vi "log analysis_gps.vi"() -> ()   [LabVIEW 2018] (continued)
0.0927,0.0768,0.1395,0.1446,5.0385,0f000001,0*5a4f325f\n\tsystem status\tnormal 2 27.900000 0 0\trobot status\t327.041164\t38.648873\t11.416000\t-0.542047\t1.417066\t-27.580040\t0.262000\t0.075000\n\t\n15:26:44.7\tlog_raw\tgps_raw\t#INSPVAXA,USB3,0,52.0,FINESTEERING,2107,282422.700,02000000,471d,15824;INS_ALIGNMENT_COMPLETE,INS_RTKFIXED,37.37047779147,126.72452855561,11.4180,22.3000,-0.1674,0.2510,0.0061,-0.538633427,1.577251598,117.409835923,0.4474,0.2945,0.5457,0.1156,0.0927,0.0768,0.1395,0.1446,5.0385,0f000001,0*702f4b29\n\tsystem status\tnormal 2 28.000000 0 0\trobot status\t327.159797\t38.571286\t11.418000\t-0.538633\t1.577252\t-27.409836\t0.344000\t-0.072000\n\t\n15:26:45.2\tlog_raw\tgps_raw\t#INSPVAXA,USB3,0,53.0,FINESTEERING,2107,282423.200,02000000,471d,15824;INS_ALIGNMENT_COMPLETE,INS_RTKFIXED,37.37047709132,126.72452988330,11.4199,22.3000,-0.1693,0.2361,0.0114,-0.484097590,1.645236384,117.249213535,0.4481,0.2944,0.5459,0.1153,0.0924,0.0769,0.1394,0.1445,5.0397,0f000001,0*1f110da8\n\tsystem status\tnormal 2 28.000000 0 0\trobot status\t327.277401\t38.493575\t11.419900\t-0.484098\t1.645236\t-27.249214\t0.366000\t-0.082000\n\t\n15:26:45.7\tlog_raw\tgps_raw\t#INSPVAXA,USB3,0,53.0,FINESTEERING,2107,282423.700,02000000,471d,15824;INS_ALIGNMENT_COMPLETE,INS_RTKFIXED,37.37047638174,126.72453122858,11.4229,22.3000,-0.1794,0.2589,0.0063,-0.583943678,1.497224393,117.186202901,0.4481,0.2944,0.5459,0.1153,0.0924,0.0769,0.1394,0.1445,5.0397,0f000001,0*d1d8ac53\n\tsystem status\tnormal 2 28.000000 0 0\trobot status\t327.396564\t38.414818\t11.422900\t-0.583944\t1.497224\t-27.186203\t0.298000\t0.020000\n\t\n15:26:46.2\tlog_raw\tgps_raw\t#INSPVAXA,USB3,0,47.5,FINESTEERING,2107,282424.200,02000000,471d,15824;INS_ALIGNMENT_COMPLETE,INS_RTKFIXED,37.37047566683,126.72453256018,11.4256,22.3000,-0.1669,0.2594,-0.0024,-0.470106549,1.538680379,117.122704089,0.4483,0.2943,0.5461,0.1150,0.0923,0.0770,0.1394,0.1445,5.0409,0f000001,0*dc6910b4\n\tsystem status\tnormal 2 28.000000 0 0\trobot status\t327.514515\t38.335469\t11.425600\t-0.470107\t1.538680\t-27.122704\t0.283000\t0.031000\n\t\n15:26:46.7\tlog_raw\tgps_raw\t#INSPVAXA,USB3,0,47.5,FINESTEERING,2107,282424.700,02000000,471d,15824;INS_ALIGNMENT_COMPLETE,INS_RTKFIXED,37.37047494841,126.72453391705,11.4289,22.3000,-0.1673,0.2511,-0.0021,-0.336586213,1.463245271,117.104928251,0.4483,0.2943,0.5461,0.1150,0.0923,0.0770,0.1394,0.1445,5.0409,0f000001,0*1c6dfd0e\n\tsystem status\tnormal 2 28.000000 0 0\trobot status\t327.634704\t38.255731\t11.428900\t-0.336586\t1.463245\t-27.104928\t0.288000\t0.027000\n\t\n15:26:47.2\tlog_raw\tgps_raw\t#INSPVAXA,USB3,0,52.5,FINESTEERING,2107,282425.200,02000000,471d,15824;INS_ALIGNMENT_COMPLETE,INS_RTKFIXED,37.37047424170,126.72453526540,11.4324,22.3000,-0.1767,0.2603,-0.0045,-0.387302146,1.336492111,117.087271319,0.4481,0.2942,0.5464,0.1148,0.0922,0.0770,0.1394,0.1445,5.0421,0f000001,0*5b1ecf9b\n\tsystem status\tnormal 2 28.000000 0 0\trobot status\t327.754139\t38.177293\t11.432400\t-0.387302\t1.336492\t-27.087271\t0.304000\t0.000000\n\t\n15:26:47.7\tlog_raw\tgps_raw\t#INSPVAXA,USB3,0,52.5,FINESTEERING,2107,282425.700,02000000,471d,15824;INS_ALIGNMENT_COMPLETE,INS_RTKFIXED,37.37047353381,126.72453661330,11.4355,22.3000,-0.1756,0.2651,-0.0041,-0.429146495,1.196465105,117.112616572,0.4481,0.2942,0.5464,0.1148,0.0922,0.0770,0.1394,0.1445,5.0421,0f000001,0*c119c68d\n\tsystem status\tnormal 2 28.000000 0 0\trobot status\t327.873534\t38.098723\t11.435500\t-0.429146\t1.196465\t-27.112617\t0.300000\t-0.005000\n\t\n15:26:48.2\tlog_raw\tgps_raw\t#INSPVAXA,USB3,0,49.0,FINESTEERING,2107,282426.200,02000000,471d,15824;INS_ALIGNMENT_COMPLETE,INS_RTKFIXED,37.37047281927,126.72453797131,11.4379,22.3000,-0.1734,0.2394,0.0077,-0.416203988,1.155690665,117.100710288,0.4473,0.2939,0.5465,0.1146,0.0922,0.0771,0.1395,0.1444,5.0432,0f000001,0*775443d5\n\tsystem status\tnormal 2 28.000000 0 0\trobot status\t327.993824\t38.019415\t11.437900\t-0.416204\t1.155691\t-27.100710\t0.298000\t-0.006000\n\t\n15:26:48.7\tlog_raw\tgps_raw\t#INSPVAXA,USB3,0,49.0,FINESTEERING,2107,282426.700,02000000,471d,15824;INS_ALIGNMENT_COMPLETE,INS_RTKFIXED,37.37047210734,126.72453930572,11.4405,22.3000,-0.1867,0.2504,0.0028,-0.209968626,1.098729863,117.099023809,0.4473,0.2939,0.5465,0.1146,0.0922,0.0771,0.1395,0.1444,5.0432,0f000001,0*f26e42b0\n\tsystem status\tnormal 2 28.000000 0 0\trobot status\t328.112024\t37.940397\t11.440500\t-0.209969\t1.098730\t-27.099024\t0.303000\t-0.001000\n\t\n15:26:49.2\tlog_raw\tgps_raw\t#INSPVAXA,USB3,0,49.0,FINESTEERING,2107,282427.200,02000000,471d,15824;INS_ALIGNMENT_COMPLETE,INS_RTKFIXED,37.37047139601,126.72454064039,11.4416,22.3000,-0.1731,0.2492,-0.0012,-0.127511151,0.940148188,117.168833754,0.4465,0.2938,0.5466,0.1144,0.0924,0.0771,0.1395,0.1444,5.0441,0f000001,0*6d877c07\n\tsystem status\tnormal 2 28.000000 0 0\trobot status\t328.230247\t37.861446\t11.441600\t-0.127511\t0.940148\t-27.168834\t0.301000\t-0.007000\n\t\n15:26:49.7\tlog_raw\tgps_raw\t#INSPVAXA,USB3,0,49.0,FINESTEERING,2107,282427.700,02000000,471d,15824;INS_ALIGNMENT_COMPLETE,INS_RTKFIXED,37.37047069525,126.72454194730,11.4442,22.3000,-0.1701,0.2495,0.0012,-0.095196200,0.956873575,117.185221868,0.4465,0.2938,0.5466,0.1144,0.0924,0.0771,0.1395,0.1444,5.0441,0f000001,0*84a20544\n\tsystem status\tnormal 2 28.000000 0 0\trobot status\t328.346010\t37.783668\t11.444200\t-0.095196\t0.956874\t-27.185222\t0.304000\t-0.005000\n\t\n15:26:50.2\tlog_raw\tgps_raw\t#INSPVAXA,USB3,0,48.5,FINESTEERING,2107,282428.200,02000000,471d,15824;INS_ALIGNMENT_COMPLETE,INS_RTKFIXED,37.37046998613,126.72454328070,11.4463,22.3000,-0.1686,0.2345,-0.0007,-0.178803832,1.054572060,117.268598245,0.4452,0.2937,0.5465,0.1143,0.0923,0.0771,0.1395,0.1444,5.0443,0f000001,0*71fff611\n\tsystem status\tnormal 2 28.000000 0 0\trobot status\t328.464121\t37.704962\t11.446300\t-0.178804\t1.054572\t-27.268598\t0.301000\t-0.003000\n\t\n15:26:50.7\tlog_raw\tgps_raw\t#INSPVAXA,USB3,0,48.5,FINESTEERING,2107,282428.700,02000000,471d,15824;INS_ALIGNMENT_COMPLETE,INS_RTKFIXED,37.37046928771,126.72454456958,11.4489,22.3000,-0.1768,0.2502,0.0012,-0.177631825,1.040630154,117.335486579,0.4452,0.2937,0.5465,0.1143,0.0923,0.0771,0.1395,0.1444,5.0443,0f000001,0*5554e59a\n\tsystem status\tnormal 2 28.000000 0 0\trobot status\t328.578288\t37.627444\t11.448900\t-0.177632\t1.040630\t-27.335487\t0.304000\t-0.005000\n\t\n15:26:51.2\tlog_raw\tgps_raw\t#INSPVAXA,USB3,0,50.5,FINESTEERING,2107,282429.200,02000000,471d,15824;INS_ALIGNMENT_COMPLETE,INS_RTKFIXED,37.37046858218,126.72454587294,11.4510,22.3000,-0.1735,0.2382,-0.0057,-0.224101923,1.178682503,117.429703451,0.4445,0.2937,0.5467,0.1141,0.0923,0.0771,0.1395,0.1444,5.0440,0f000001,0*7240883e\n\tsystem status\tnormal 2 28.000000 0 0\trobot status\t328.693737\t37.549136\t11.451000\t-0.224102\t1.178683\t-27.429703\t0.303000\t-0.014000\n\t\n15:26:51.7\tlog_raw\tgps_raw\t#INSPVAXA,USB3,0,50.5,FINESTEERING,2107,282429.700,02000000,471d,15824;INS_ALIGNMENT_COMPLETE,INS_RTKFIXED,37.37046786468,126.72454718856,11.4534,22.3000,-0.1761,0.2406,-0.0007,-0.208083401,1.502280948,117.509973758,0.4445,0.2937,0.5467,0.1141,0.0923,0.0771,0.1395,0.1444,5.0440,0f000001,0*e6f82928\n\tsystem status\tnormal 2 28.000000 0 0\trobot status\t328.810273\t37.469500\t11.453400\t-0.208083\t1.502281\t-27.509974\t0.294000\t-0.015000\n\t\n15:26:52.2\tlog_raw\tgps_raw\t#INSPVAXA,USB3,0,50.5,FINESTEERING,2107,282430.200,02000000,471d,15824;INS_ALIGNMENT_COMPLETE,INS_RTKFIXED,37.37046713454,126.72454853223,11.4571,22.3000,-0.1871,0.2437,0.0106,-0.235134263,1.524805783,117.657150999,0.4436,0.2937,0.5464,0.1140,0.0923,0.0770,0.1395,0.1444,5.0440,0f000001,0*40fb5b15\n\tsystem status\tnormal 2 28.000000 0 0\trobot status\t328.929293\t37.388461\t11.457100\t-0.235134\t1.524806\t-27.657151\t0.302000\t-0.003000\n\t\n15:26:52.7\tlog_raw\tgps_raw\t#INSPVAXA,USB3,0,50.5,FINESTEERING,2107,282430.700,02000000,471d,15824;INS_ALIGNMENT_COMPLETE,INS_RTKFIXED,37.37046640925,126.72454987215,11.4613,22.3000,-0.1820,0.2459,0.0096,-0.221423575,1.571464765,117.878951435,0.4436,0.2937,0.5464,0.1140,0.0923,0.0770,0.1395,0.1444,5.0440,0f000001,0*a08ac800\n\tsystem status\tnormal 2 28.000000 0 0\trobot status\t329.047981\t37.307960\t11.461300\t-0.221424\t1.571465\t-27.878951\t0.302000\t-0.009000\n\t\n15:26:53.2\tlog_raw\tgps_raw\t#INSPVAXA,USB3,0,50.5,FINESTEERING,2107,282431.200,02000000,471d,15824;INS_ALIGNMENT_COMPLETE,INS_RTKFIXED,37.37046567554,126.72455119637,11.4651,22.3000,-0.1719,0.2427,0.0197,-0.166037834,1.730159075,118.106300451,0.4429,0.2934,0.5460,0.1140,0.0922,0.0770,0.1395,0.1444,5.0446,0f000001,0*c5fa0f53\n\tsystem status\tnormal 2 28.000000 0 0\trobot status\t329.165278\t37.226525\t11.465100\t-0.166038\t1.730159\t-28.106300\t0.300000\t-0.008000\n\t\n15:26:53.7\tlog_raw\tgps_raw\t#INSPVAXA,USB3,0,50.5,FINESTEERING,2107,282431.700,02000000,471d,15824;INS_ALIGNMENT_COMPLETE,INS_RTKFIXED,37.37046493957,126.72455254233,11.4688,22.3000,-0.1743,0.2458,0.0116,-0.329831590,1.590746400,118.317737739,0.4429,0.2934,0.5460,0.1140,0.0922,0.0770,0.1395,0.1444,5.0446,0f000001,0*f79436a0\n\tsystem status\tnormal 2 28.000000 0 0\trobot status\t329.284501\t37.144839\t11.468800\t-0.329832\t1.590746\t-28.317738\t0.295000\t-0.010000\n\t\n15:26:54.2\tlog_raw\tgps_raw\t#INSPVAXA,USB3,0,51.5,FINESTEERING,2107,282432.200,02000000,471d,15824;INS_ALIGNMENT_COMPLETE,INS_RTKFIXED,37.37046419639,126.72455389364,11.4732,22.3000,-0.1776,0.2446,0.0108,-0.495947229,1.503105474,118.571137499,0.4424,0.2936,0.5455,0.1139,0.0922,0.0769,0.1394,0.1444,5.0458,0f000001,0*be714efa\n\tsystem status\tnormal 2 28.000000 0 0\trobot status\t329.404198\t37.062353\t11.473200\t-0.495947\t1.503105\t-28.571137\t0.296000\t-0.015000\n\t\n15:26:54.7\tlog_raw\tgps_raw\t#INSPVAXA,USB3,0,51.5,FINESTEERING,2107,282432.700,02000000,471d,15824;INS_ALIGNMENT_COMPLETE,INS_RTKFIXED,37.37046345455,126.72455522466,11.4784,22.3000,-0.1781,0.2428,0.0084,-0.542024872,1.613123448,118.821399108,0.4424,0.2936,0.5455,0.1139,0.0922,0.0769,0.1394,0.1444,5.0458,0f000001,0*f6f3aed6\n\tsystem status\tnormal 2 28.000000 0 0\trobot status\t329.522097\t36.980016\t11.478400\t-0.542025\t1.613123\t-28.821399\t0.295000\t-0.017000\n\t\n15:26:55.2\tlog_raw\tgps_raw\t#INSPVAXA,USB3,0,50.0,FINESTEERING,2107,282433.200,02000000,471d,15824;INS_ALIGNMENT_COMPLETE,INS_RTKFIXED,37.37046270348,126.72455655878,11.4838,22.3000,-0.1795,0.2457,0.0085,-0.467602875,1.636327980,119.061626525,0.4415,0.2938,0.5451,0.1139,0.0923,0.0769,0.1394,0.1444,5.0472,0f000001,0*8d27345e\n\tsystem status\tnormal 2 28.000000 0 0\trobot status\t329.640271\t36.896654\t11.483800\t-0.467603\t1.636328\t-29.061627\t0.302000\t-0.014000\n\t\n15:26:55.7\tlog_raw\tgps_raw\t#DUALANTENNAHEADINGA,USB3,0,50.0,FINESTEERING,2107,282433.700,02000000,d426,15824;SOL_COMPUTED,NARROW_FLOAT,-1.000000000,131.824783325,-60.644287109,0.0,360.000000000,180.000000000,\"631T\",16,7,7,6,04,00,20,03*5e82c6fa\n\tsystem status\tnormal 2 28.000000 0 0\trobot status\t329.757799\t36.814629\t11.489300\t-0.433063\t1.678880\t-29.334865\t0.303000\t-0.012000\n\t\n15:26:56.2\tlog_raw\tgps_raw\t#INSPVAXA,USB3,0,51.0,FINESTEERING,2107,282434.200,02000000,471d,15824;INS_ALIGNMENT_COMPLETE,INS_RTKFIXED,37.37046121342,126.72455921489,11.4947,22.3000,-0.1798,0.2490,0.0001,-0.438174613,1.842528382,119.643730072,0.4410,0.2940,0.5447,0.1139,0.0923,0.0769,0.1394,0.1443,5.0488,0f000001,0*2736b416\n\tsystem status\tnormal 2 28.000000 0 0\trobot status\t329.875545\t36.731271\t11.494700\t-0.438175\t1.842528\t-29.643730\t0.309000\t-0.015000\n\t\n15:26:56.7\tlog_raw\tgps_raw\t#DUALANTENNAHEADINGA,USB3,0,51.0,FINESTEERING,2107,282434.700,02000000,d426,15824;SOL_COMPUTED,NARROW_FLOAT,-1.000000000,123.396003723,-59.946563721,0.0,360.000000000,180.000000000,\"631T\",18,7,7,6,04,00,20,03*e2309186\n\tsystem status\tnormal 2 28.000000 0 0\trobot status\t329.993174\t36.646447\t11.500400\t-0.411549\t1.662187\t-29.943410\t0.300000\t-0.011000\n\t\n15:26:57.2\tlog_raw\tgps_raw\t#INSPVAXA,USB3,0,52.0,FINESTEERING,2107,282435.200,02000000,471d,15824;INS_ALIGNMENT_COMPLETE,INS_RTKFIXED,37.37045967232,126.72456187341,11.5062,22.3000,-0.1775,0.2335,0.0126,-0.320080910,1.572819973,120.246717938,0.4403,0.2940,0.5441,0.1137,0.0923,0.0768,0.1394,0.1443,5.0504,0f000001,0*2715df5d\n\tsystem status\tnormal 2 28.000000 0 0\trobot status\t330.111033\t36.560223\t11.506200\t-0.320081\t1.572820\t-30.246718\t0.290000\t-0.019000\n\t\n15:26:57.7\tlog_raw\tgps_raw\t#INSPVAXA,USB3,0,52.0,FINESTEERING,2107,282435.700,02000000,471d,15824;INS_ALIGNMENT_COMPLETE,INS_RTKFIXED,37.37045891592,126.72456315232,11.5133,22.3000,-0.1801,0.2388,0.0143,-0.294831475,1.595184630,120.686846518,0.4403,0.2940,0.5441,0.1137,0.0923,0.0768,0.1394,0.1443,5.0504,0f000001,0*d40acedf\n\tsystem status\tnormal 2 28.000000 0 0\trobot status\t330.224316\t36.476270\t11.513300\t-0.294831\t1.595185\t-30.686847\t0.300000\t-0.018000\n\t\n15:26:58.2\tlog_raw\tgps_raw\t#DUALANTENNAHEADINGA,USB3,0,49.0,FINESTEERING,2107,282436.200,02000000,d426,15824;SOL_COMPUTED,L1_FLOAT,-1.000000000,106.640296936,-71.318817139,0.0,360.000000000,180.000000000,\"631T\",16,6,6,6,04,00,20,02*b4f0dd4d\n\tsystem status\tnormal 2 28.000000 0 0\trobot status\t330.338646\t36.390312\t11.520900\t-0.272505\t1.410764\t-31.156863\t0.335000\t0.034000\n\t\n15:26:58.7\tlog_raw\tgps_raw\t#INSPVAXA,USB3,0,49.0,FINESTEERING,2107,282436.700,02000000,471d,15824;INS_ALIGNMENT_COMPLETE,INS_RTKFIXED,37.37045734595,126.72456573410,11.5280,22.3000,-0.1935,0.2298,0.0134,-0.155063449,1.404576364,121.642005651,0.4395,0.2941,0.5437,0.1137,0.0923,0.0768,0.1394,0.1443,5.0520,0f000001,0*bb2e31e4\n\tsystem status\tnormal 2 28.000000 0 0\trobot status\t330.453006\t36.302018\t11.528000\t-0.155063\t1.404576\t-31.642006\t0.365000\t0.096000\n\t\n15:26:59.2\tlog_raw\tgps_raw\t#DUALANTENNAHEADINGA,USB3,0,50.0,FINESTEERING,2107,282437.200,02000000,d426,15824;SOL_COMPUTED,L1_FLOAT,-1.000000000,96.910743713,-72.679077148,0.0,360.000000000,180.000000000,\"631T\",19,6,6,6,04,00,20,02*8360ff91\n\tsystem status\tnormal 2 28.000000 0 0\trobot status\t330.566267\t36.213333\t11.534500\t-0.164952\t1.430283\t-32.232703\t0.293000\t-0.018000\n\t\n15:26:59.7\tlog_raw\tgps_raw\t#INSPVAXA,USB3,0,50.0,FINESTEERING,2107,282437.700,02000000,471d,15824;INS_ALIGNMENT_COMPLETE,INS_RTKFIXED,37.37045573344,126.72456827532,11.5401,22.3000,-0.1925,0.2230,0.0039,-0.101664053,1.395103847,122.819960781,0.4390,0.2940,0.5434,0.1136,0.0923,0.0768,0.1393,0.1443,5.0536,0f000001,0*7037bf1b\n\tsystem status\tnormal 2 28.000000 0 0\trobot status\t330.678103\t36.123046\t11.540100\t-0.101664\t1.395104\t-32.819961\t0.253000\t-0.080000\n\t\n15:27:00.2\tlog_raw\tgps_raw\t#INSPVAXA,USB3,0,50.0,FINESTEERING,2107,282438.200,02000000,471d,15824;INS_ALIGNMENT_COMPLETE,INS_RTKFIXED,37.37045491060,126.72456953243,11.5455,22.3000,-0.2008,0.2357,0.0053,0.014344275,1.355437453,123.346628191,0.4390,0.2941,0.5434,0.1137,0.0924,0.0768,0.1393,0.1442,5.0551,0f000001,0*dff132ba\n\tsystem status\tnormal 2 28.000000 0 0\trobot status\t330.789456\t36.031719\t11.545500\t0.014344\t1.355437\t-33.346628\t0.238000\t-0.107000\n\t\n15:27:00.7\tlog_raw\tgps_raw\t#DUALANTENNAHEADINGA,USB3,0,50.0,FINESTEERING,2107,282438.700,02000000,d426,15824;SOL_COMPUTED,L1_FLOAT,-1.000000000,88.413047791,-71.788269043,0.0,360.000000000,180.000000000,\"631T\",18,6,6,6,04,00,20,02*2c629dff\n\tsystem status\tnormal 2 28.000000 0 0\trobot status\t330.900070\t35.941719\t11.550100\t-0.061999\t1.261204\t-33.976038\t0.479000\t0.250000\n\t\n15:27:01.2\tlog_raw\tgps_raw\t#INSPVAXA,USB3,0,50.0,FINESTEERING,2107,282439.200,02000000,471d,15824;INS_ALIGNMENT_COMPLETE,INS_RTKFIXED,37.37045327515,126.72457200687,11.5547,22.3000,-0.1947,0.2312,0.0176,0.007839665,1.196473150,124.504878880,0.4394,0.2943,0.5435,0.1138,0.0925,0.0768,0.1393,0.1442,5.0565,0f000001,0*62131131\n\tsystem status\tnormal 2 28.000000 0 0\trobot status\t331.008638\t35.850200\t11.554700\t0.007840\t1.196473\t-34.504879\t0.366000\t0.072000\n\t\n15:27:01.7\tlog_raw\tgps_raw\t#INSPVAXA,USB3,0,50.0,FINESTEERING,2107,282439.700,02000000,471d,15824;INS_ALIGNMENT_COMPLETE,INS_RTKFIXED,37.37045245095,126.72457319458,11.5591,22.3000,-0.1909,0.2308,0.0250,0.014196005,1.345300679,124.975912941,0.4394,0.2943,0.5435,0.1138,0.0925,0.0768,0.1393,0.1442,5.0565,0f000001,0*c01a2c95\n\tsystem status\tnormal 2 28.000000 0 0\trobot status\t331.113843\t35.758723\t11.559100\t0.014196\t1.345301\t-34.975913\t0.284000\t-0.034000\n\t\n15:27:02.2\tlog_raw\tgps_raw\t#DUALANTENNAHEADINGA,USB3,0,50.5,FINESTEERING,2107,282440.200,02000000,d426,15824;SOL_COMPUTED,L1_FLOAT,-1.000000000,104.733528137,-71.981353760,0.0,360.000000000,180.000000000,\"631T\",16,6,6,6,04,00,20,02*496cf2b0\n\tsystem status\tnormal 2 28.000000 0 0\trobot status\t331.219713\t35.666735\t11.563700\t0.016944\t1.696880\t-35.321999\t0.302000\t-0.004000\n\t\n15:27:02.7\tlog_raw\tgps_raw\t#INSPVAXA,USB3,0,50.5,FINESTEERING,2107,282440.700,02000000,471d,15824;INS_ALIGNMENT_COMPLETE,INS_RTKFIXED,37.37045078135,126.72457562131,11.5665,22.3000,-0.1912,0.2138,0.0152,-0.119688285,1.522549253,125.693506579,0.4396,0.2937,0.5434,0.1139,0.0925,0.0768,0.1392,0.1442,5.0578,0f000001,0*ce1f2ed1\n\tsystem status\tnormal 2 28.000000 0 0\trobot status\t331.328799\t35.573414\t11.566500\t-0.119688\t1.522549\t-35.693507\t0.344000\t0.082000\n\t\n15:27:03.2\tlog_raw\tgps_raw\t#DUALANTENNAHEADINGA,USB3,0,53.0,FINESTEERING,2107,282441.200,02000000,d426,15824;SOL_COMPUTED,L1_FLOAT,-1.000000000,98.119506836,-70.068420410,0.0,360.000000000,180.000000000,\"631T\",15,6,6,6,04,00,20,02*34737370\n\tsystem status\tnormal 2 28.000000 0 0\trobot status\t331.432619\t35.480504\t11.569000\t-0.082738\t1.498113\t-36.012425\t0.247000\t-0.082000\n\t\n15:27:03.7\tlog_raw\tgps_raw\t#INSPVAXA,USB3,0,53.0,FINESTEERING,2107,282441.700,02000000,471d,15824;INS_ALIGNMENT_COMPLETE,INS_RTKFIXED,37.37044907161,126.72457798223,11.5726,22.3000,-0.1948,0.2179,0.0112,0.019648441,1.409240811,126.353403085,0.4397,0.2935,0.5431,0.1139,0.0925,0.0768,0.1391,0.1441,5.0591,0f000001,0*4c7348f3\n\tsystem status\tnormal 2 28.000000 0 0\trobot status\t331.537926\t35.383651\t11.572600\t0.019648\t1.409241\t-36.353403\t0.229000\t-0.093000\n\t\n15:27:04.2\tlog_raw\tgps_raw\t#DUALANTENNAHEADINGA,USB3,0,53.0,FINESTEERING,2107,282442.200,02000000,d426,15824;SOL_COMPUTED,L1_FLOAT,-1.000000000,135.735549927,-62.905853271,0.0,360.000000000,180.000000000,\"631T\",15,6,6,6,04,00,20,02*7d1a323e\n\tsystem status\tnormal 2 28.000000 0 0\trobot status\t331.643745\t35.286306\t11.577800\t0.040624\t1.148557\t-36.777461\t0.347000\t0.059000\n\t\n15:27:04.7\tlog_raw\tgps_raw\t#DUALANTENNAHEADINGA,USB3,0,53.0,FINESTEERING,2107,282442.700,02000000,d426,15824;SOL_COMPUTED,L1_FLOAT,-1.000000000,139.850036621,-63.364013672,0.0,360.000000000,180.000000000,\"631T\",16,6,6,6,04,00,20,02*201824d6\n\tsystem status\tnormal 2 28.000000 0 0\trobot status\t331.748506\t35.190562\t11.582000\t-0.114390\t1.160307\t-37.256257\t0.280000\t-0.049000\n\t\n15:27:05.2\tlog_raw\tgps_raw\t#INSPVAXA,USB3,0,51.0,FINESTEERING,2107,282443.200,02000000,471d,15824;INS_ALIGNMENT_COMPLETE,INS_RTKFIXED,37.37044646413,126.72458151712,11.5864,22.3000,-0.1973,0.2015,0.0164,-0.221608077,1.394071169,127.627895652,0.4382,0.2942,0.5425,0.1139,0.0929,0.0768,0.1390,0.1440,5.0619,0f000001,0*d0821dfc\n\tsystem status\tnormal 2 28.000000 0 0\trobot status\t331.851040\t35.094249\t11.586400\t-0.221608\t1.394071\t-37.627896\t0.338000\t0.046000\n\t\n15:27:05.7\tlog_raw\tgps_raw\t#DUALANTENNAHEADINGA,USB3,0,51.0,FINESTEERING,2107,282443.700,02000000,d426,15824;SOL_COMPUTED,NARROW_FLOAT,-1.000000000,112.599952698,-57.933044434,0.0,360.000000000,180.000000000,\"631T\",15,6,6,6,04,00,20,03*0a41350b\n\tsystem status\tnormal 2 28.000000 0 0\trobot status\t331.952897\t34.994891\t11.593000\t-0.249153\t1.572965\t-38.005093\t0.379000\t0.102000\n\t\n15:27:06.2\tlog_raw\tgps_raw\t#DUALANTENNAHEADINGA,USB3,0,52.5,FINESTEERING,2107,282444.200,02000000,d426,15824;SOL_COMPUTED,L1_FLOAT,-1.000000000,94.401931763,-65.202850342,0.0,360.000000000,180.000000000,\"631T\",17,6,6,6,04,00,20,03*e210f1e8\n\tsystem status\tnormal 2 28.000000 0 0\trobot status\t332.052872\t34.895652\t11.599300\t-0.212433\t1.862768\t-38.371437\t0.256000\t-0.080000\n\t\n15:27:06.7\tlog_raw\tgps_raw\t#INSPVAXA,USB3,0,52.5,FINESTEERING,2107,282444.700,02000000,471d,15824;INS_ALIGNMENT_COMPLETE,INS_RTKFIXED,37.37044378367,126.72458489519,11.6040,22.3000,-0.1971,0.2104,0.0118,-0.197880099,2.000562987,128.752453378,0.4375,0.2942,0.5421,0.1140,0.0930,0.0767,0.1389,0.1439,5.0634,0f000001,0*c33b9934\n\tsystem status\tnormal 2 28.000000 0 0\trobot status\t332.150264\t34.796747\t11.604000\t-0.197880\t2.000563\t-38.752453\t0.332000\t0.027000\n\t\n15:27:07.2\tlog_raw\tgps_raw\t#INSPVAXA,USB3,0,52.0,FINESTEERING,2107,282445.200,02000000,471d,15824;INS_ALIGNMENT_COMPLETE,INS_RTKFIXED,37.37044286692,126.72458603367,11.6088,22.3000,-0.1958,0.2105,0.0125,-0.182257004,1.882197193,129.119511082,0.4372,0.2942,0.5419,0.1140,0.0930,0.0767,0.1387,0.1438,5.0651,0f000001,0*e6286548\n\tsystem status\tnormal 2 28.000000 0 0\trobot status\t332.251109\t34.694998\t11.608800\t-0.182257\t1.882197\t-39.119511\t0.284000\t-0.033000\n\t\n15:27:07.7\tlog_raw\tgps_raw\t#INSPVAXA,USB3,0,52.0,FINESTEERING,2107,282445.700,02000000,471d,15824;INS_ALIGNMENT_COMPLETE,INS_RTKFIXED,37.37044196596,126.72458716165,11.6139,22.3000,-0.1860,0.1986,0.0135,-0.288793449,1.691261499,129.571848658,0.4372,0.2942,0.5419,0.1140,0.0930,0.0767,0.1387,0.1438,5.0651,0f000001,0*93ea3f3c\n\tsystem status\tnormal 2 28.000000 0 0\trobot status\t332.351024\t34.595001\t11.613900\t-0.288793\t1.691261\t-39.571849\t0.238000\t-0.092000\n\t\n15:27:08.2\tlog_raw\tgps_raw\t#INSPVAXA,USB3,0,49.5,FINESTEERING,2107,282446.200,02000000,471d,15824;INS_ALIGNMENT_COMPLETE,INS_RTKFIXED,37.37044104802,126.72458827290,11.6191,22.3000,-0.2036,0.2086,0.0326,-0.314944845,1.597002545,130.029060418,0.4370,0.2950,0.5417,0.1141,0.0931,0.0767,0.1386,0.1437,5.0666,0f000001,0*166a3618\n\tsystem status\tnormal 2 28.000000 0 0\trobot status\t332.449456\t34.493120\t11.619100\t-0.314945\t1.597003\t-40.029060\t0.265000\t-0.068000\n\t\n15:27:08.7\tlog_raw\tgps_raw\t#DUALANTENNAHEADINGA,USB3,0,49.5,FINESTEERING,2107,282446.700,02000000,d426,15824;SOL_COMPUTED,L1_FLOAT,-1.000000000,72.571334839,-68.740661621,0.0,360.000000000,180.000000000,\"631T\",16,6,6,6,04,00,20,02*f8abca53\n\tsystem status\tnormal 2 28.000000 0 0\trobot status\t332.546590\t34.388271\t11.623500\t-0.257290\t1.459465\t-40.450598\t0.287000\t-0.037000\n\t\n15:27:09.2\tlog_raw\tgps_raw\t#DUALANTENNAHEADINGA,USB3,0,51.0,FINESTEERING,2107,282447.200,02000000,d426,15824;SOL_COMPUTED,L1_FLOAT,-1.000000000,47.042289734,-21.824493408,0.0,80.520454407,171.226654053,\"631T\",17,6,6,6,04,00,20,02*c2df237f\n\tsystem status\tnormal 2 28.000000 0 0\trobot status\t332.644198\t34.281714\t11.627900\t-0.223387\t1.426203\t-40.898796\t0.297000\t-0.021000\n\t\n15:27:09.7\tlog_raw\tgps_raw\t#DUALANTENNAHEADINGA,USB3,0,51.0,FINESTEERING,2107,282447.700,02000000,d426,15824;SOL_COMPUTED,L1_FLOAT,-1.000000000,47.179916382,-22.115081787,0.0,81.568397522,172.185485840,\"631T\",16,6,6,6,04,00,20,02*ed165946\n\tsystem status\tnormal 2 28.000000 0 0\trobot status\t332.740064\t34.175121\t11.632300\t-0.181305\t1.536050\t-41.293429\t0.230000\t-0.140000\n\t\n15:27:10.2\tlog_raw\tgps_raw\t#DUALANTENNAHEADINGA,USB3,0,50.0,FINESTEERING,2107,282448.200,02000000,d426,15824;SOL_COMPUTED,L1_FLOAT,-1.000000000,62.731056213,-70.065948486,0.0,206.330291748,71.296012878,\"631T\",14,6,6,6,04,00,20,02*363416aa\n\tsystem status\tnormal 2 28.000000 0 0\trobot status\t332.834657\t34.068208\t11.636100\t-0.115686\t1.476151\t-41.714557\t0.390000\t0.115000\n\t\n15:27:10.7\tlog_raw\tgps_raw\t#DUALANTENNAHEADINGA,USB3,0,50.0,FINESTEERING,2107,282448.700,02000000,d426,15824;SOL_COMPUTED,L1_FLOAT,-1.000000000,63.022411346,-70.363861084,0.0,209.852844238,71.028411865,\"631T\",14,6,6,6,04,00,20,02*916b79b1\n\tsystem status\tnormal 2 28.000000 0 0\trobot status\t332.929227\t33.960423\t11.639600\t-0.032914\t1.412595\t-42.067296\t0.272000\t-0.049000\n\t\n15:27:11.2\tlog_raw\tgps_raw\t#INSPVAXA,USB3,0,52.0,FINESTEERING,2107,282449.200,02000000,471d,15824;INS_ALIGNMENT_COMPLETE,INS_RTKFIXED,37.37043526808,126.72459474033,11.6436,22.3000,-0.2045,0.1792,0.0240,0.090566175,1.487884690,132.369305266,0.4363,0.2959,0.5410,0.1143,0.0932,0.0767,0.1382,0.1433,5.0710,0f000001,0*e0923cb2\n\tsystem status\tnormal 2 28.000000 0 0\trobot status\t333.022331\t33.851613\t11.643600\t0.090566\t1.487885\t-42.369305\t0.345000\t0.066000\n\t\n15:27:11.7\tlog_raw\tgps_raw\t#DUALANTENNAHEADINGA,USB3,0,52.0,FINESTEERING,2107,282449.700,02000000,d426,15824;SOL_COMPUTED,L1_FLOAT,-1.000000000,47.736373901,-41.870452881,0.0,87.065238953,101.863716125,\"631T\",13,6,6,6,04,00,20,02*14df9d16\n\tsystem status\tnormal 2 28.000000 0 0\trobot status\t333.114293\t33.743890\t11.647700\t0.044999\t1.426997\t-42.670199\t0.294000\t-0.011000\n\t\n15:27:12.2\tlog_raw\tgps_raw\t#DUALANTENNAHEADINGA,USB3,0,53.5,FINESTEERING,2107,282450.200,02000000,d426,15824;SOL_COMPUTED,L1_FLOAT,-1.000000000,51.328735352,-27.176086426,0.0,71.032249451,148.623870850,\"631T\",13,6,6,6,04,00,20,02*70d3e876\n\tsystem status\tnormal 2 28.000000 0 0\trobot status\t333.205049\t33.634125\t11.650600\t0.240136\t1.430661\t-42.939350\t0.307000\t-0.007000\n\t\n15:27:12.7\tlog_raw\tgps_raw\t#DUALANTENNAHEADINGA,USB3,0,53.5,FINESTEERING,2107,282450.700,02000000,d426,15824;SOL_COMPUTED,L1_FLOAT,-1.000000000,51.277191162,-27.081176758,0.0,70.920402527,148.848937988,\"631T\",13,6,6,6,04,00,20,02*7b58cb2d\n\tsystem status\tnormal 2 28.000000 0 0\trobot status\t333.298460\t33.521084\t11.652900\t0.368602\t1.372850\t-43.254713\t0.294000\t-0.011000\n\t\n15:27:13.2\tlog_raw\tgps_raw\t#DUALANTENNAHEADINGA,USB3,0,52.5,FINESTEERING,2107,282451.200,02000000,d426,15824;SOL_COMPUTED,L1_FLOAT,-1.000000000,57.890838623,-57.911682129,0.0,124.624069214,87.193580627,\"631T\",15,6,6,6,04,00,20,02*079d44e7\n\tsystem status\tnormal 2 28.000000 0 0\trobot status\t333.389705\t33.410958\t11.655500\t0.274163\t1.507707\t-43.538741\t0.296000\t-0.007000\n\t\n15:27:13.7\tlog_raw\tgps_raw\t#DUALANTENNAHEADINGA,USB3,0,52.5,FINESTEERING,2107,282451.700,02000000,d426,15824;SOL_COMPUTED,L1_FLOAT,-1.000000000,57.663475037,-57.904479980,0.0,124.210479736,87.412086487,\"631T\",14,6,6,6,04,00,20,03*cca5b843\n\tsystem status\tnormal 2 28.000000 0 0\trobot status\t333.482165\t33.298901\t11.658400\t0.177384\t1.428253\t-43.810446\t0.296000\t-0.012000\n\t\n15:27:14.2\tlog_raw\tgps_raw\t#DUALANTENNAHEADINGA,USB3,0,52.0,FINESTEERING,2107,282452.200,02000000,d426,15824;SOL_COMPUTED,L1_FLOAT,-1.000000000,54.869430542,-44.105773926,0.0,97.000511169,118.565223694,\"631T\",14,6,6,6,04,00,20,02*875da1f2\n\tsystem status\tnormal 2 28.000000 0 0\trobot status\t333.573111\t33.186729\t11.660700\t0.187302\t1.410985\t-44.065241\t0.300000\t-0.010000\n\t\n15:27:14.7\tlog_raw\tgps_raw\t#DUALANTENNAHEADINGA,USB3,0,52.0,FINESTEERING,2107,282452.700,02000000,d426,15824;SOL_COMPUTED,L1_FLOAT,-1.000000000,55.240604401,-44.770904541,0.0,98.983810425,117.544937134,\"631T\",14,6,6,6,04,00,20,02*e9f54d5e\n\tsystem status\tnormal 2 28.000000 0 0\trobot status\t333.662065\t33.075313\t11.662300\t0.284712\t1.506154\t-44.271764\t0.300000\t0.003000\n\t\n15:27:15.2\tlog_raw\tgps_raw\t#DUALANTENNAHEADINGA,USB3,0,50.5,FINESTEERING,2107,282453.200,02000000,d426,15824;SOL_COMPUTED,L1_FLOAT,-1.000000000,53.051345825,-30.869628906,0.0,85.964683533,159.088867188,\"631T\",12,6,6,6,04,00,20,02*9757b4ba\n\tsystem status\tnormal 2 28.000000 0 0\trobot status\t333.749907\t32.964151\t11.664300\t0.398079\t1.550212\t-44.520288\t0.304000\t-0.002000\n\t\n15:27:15.7\tlog_raw\tgps_raw\t#DUALANTENNAHEADINGA,USB3,0,50.5,FINESTEERING,2107,282453.700,02000000,d426,15824;SOL_COMPUTED,L1_FLOAT,-1.000000000,53.156692505,-31.481872559,0.0,86.806381226,157.845855713,\"631T\",12,6,6,6,04,00,20,02*cbe10416\n\tsystem status\tnormal 2 28.000000 0 0\trobot status\t333.838695\t32.853047\t11.667600\t0.324248\t1.452403\t-44.787555\t0.299000\t-0.003000\n\t\n15:27:16.2\tlog_raw\tgps_raw\t#DUALANTENNAHEADINGA,USB3,0,52.0,FINESTEERING,2107,282454.200,02000000,d426,15824;SOL_COMPUTED,L1_FLOAT,-1.000000000,52.780334473,-53.877258301,0.0,130.208221436,141.251815796,\"631T\",14,6,6,6,04,00,20,02*fcced73a\n\tsystem status\tnormal 2 28.000000 0 0\trobot status\t333.930474\t32.739277\t11.670000\t0.290150\t1.254826\t-44.992673\t0.300000\t0.000000\n\t\n15:27:16.7\tlog_raw\tgps_raw\t#DUALANTENNAHEADINGA,USB3,0,52.0,FINESTEERING,2107,282454.700,02000000,d426,15824;SOL_COMPUTED,L1_FLOAT,-1.000000000,52.636894226,-53.647705078,0.0,129.656005859,142.158767700,\"631T\",13,6,6,6,04,00,20,02*0d3c93fe\n\tsystem status\tnormal 2 28.000000 0 0\trobot status\t334.021378\t32.628145\t11.671800\t0.255531\t1.219635\t-45.071871\t0.297000\t0.001000\n\t\n15:27:17.2\tlog_raw\tgps_raw\t\tsystem status\tnormal 2 28.000000 0 0\trobot status\t334.114386\t32.514788\t11.673700\t0.196509\t1.072827\t-45.139294\t0.294000\t0.012000\n\t\n15:27:17.7\tlog_raw\tgps_raw\t#DUALANTENNAHEADINGA,USB3,0,51.5,FINESTEERING,2107,282455.700,02000000,d426,15824;SOL_COMPUTED,L1_FLOAT,-1.000000000,51.760696411,-51.082702637,0.0,133.844039917,173.444122314,\"631T\",14,6,6,6,04,00,20,02*f8aac9e6\n\tsystem status\tnormal 2 28.000000 0 0\trobot status\t334.206369\t32.399036\t11.675200\t0.326858\t0.794167\t-45.162591\t0.295000\t0.004000\n\t\n15:27:18.2\tlog_raw\tgps_raw\t#DUALANTENNAHEADINGA,USB3,0,53.5,FINESTEERING,2107,282456.200,02000000,d426,15824;SOL_COMPUTED,L1_FLOAT,-1.000000000,51.028530121,-49.821136475,0.0,115.512840271,104.671615601,\"631T\",14,6,6,6,04,00,20,02*e59d7854\n\tsystem status\tnormal 2 28.000000 0 0\trobot status\t334.298520\t32.282316\t11.675800\t0.467199\t0.679863\t-45.205921\t0.299000\t0.005000\n\t\n15:27:18.7\tlog_raw\tgps_raw\t#DUALANTENNAHEADINGA,USB3,0,53.5,FINESTEERING,2107,282456.700,02000000,d426,15824;SOL_COMPUTED,L1_FLOAT,-1.000000000,51.237274170,-50.023620605,0.0,116.616584778,104.545890808,\"631T\",13,6,6,6,04,00,20,02*1b2f8a7d\n\tsystem status\tnormal 2 28.000000 0 0\trobot status\t334.388515\t32.167668\t11.676700\t0.570279\t0.764132\t-45.179052\t0.300000\t0.008000\n\t\n15:27:19.2\tlog_raw\tgps_raw\t#DUALANTENNAHEADINGA,USB3,0,53.0,FINESTEERING,2107,282457.200,02000000,d426,15824;SOL_COMPUTED,L1_FLOAT,-1.000000000,50.694931030,-44.774475098,0.0,121.998092651,121.907302856,\"631T\",13,6,6,6,04,00,20,02*d464c5aa\n\tsystem status\tnormal 2 28.000000 0 0\trobot status\t334.479714\t32.052386\t11.679100\t0.588296\t0.790634\t-45.211656\t0.303000\t0.014000\n\t\n15:27:19.7\tlog_raw\tgps_raw\t#DUALANTENNAHEADINGA,USB3,0,53.0,FINESTEERING,2107,282457.700,02000000,d426,15824;SOL_COMPUTED,L1_FLOAT,-1.000000000,50.592933655,-45.348266602,0.0,122.468826294,120.254112244,\"631T\",13,6,6,6,04,00,20,02*d8abe33e\n\tsystem status\tnormal 2 28.000000 0 0\trobot status\t334.571585\t31.940016\t11.682700\t0.367314\t1.055246\t-45.034349\t0.307000\t0.025000\n\t\n15:27:20.2\tlog_raw\tgps_raw\t#DUALANTENNAHEADINGA,USB3,0,53.0,FINESTEERING,2107,282458.200,02000000,d426,15824;SOL_COMPUTED,L1_FLOAT,-1.000000000,49.797100067,-45.644378662,0.0,104.331756592,110.018707275,\"631T\",15,6,6,6,04,00,20,02*7b675054\n\tsystem status\tnormal 2 27.900000 0 0\trobot status\t334.660650\t31.830333\t11.685400\t0.359168\t1.421814\t-44.643158\t0.485000\t-0.240000\n\t\n15:27:20.7\tlog_raw\tgps_raw\t#DUALANTENNAHEADINGA,USB3,0,53.0,FINESTEERING,2107,282458.700,02000000,d426,15824;SOL_COMPUTED,L1_FLOAT,-1.000000000,50.209892273,-46.350616455,0.0,106.050132751,108.550285339,\"631T\",15,6,6,6,04,00,20,02*c27fecdc\n\tsystem status\tnormal 2 27.900000 0 0\trobot status\t334.750187\t31.721037\t11.687000\t0.342961\t1.518131\t-44.190312\t0.276000\t0.053000\n\t\n15:27:21.2\tlog_raw\tgps_raw\t#DUALANTENNAHEADINGA,USB3,0,49.5,FINESTEERING,2107,282459.200,02000000,d426,15824;SOL_COMPUTED,L1_FLOAT,-1.000000000,51.845520020,-58.692413330,0.0,123.868484497,115.955833435,\"631T\",15,5,5,5,04,00,20,03*67457323\n\tsystem status\tnormal 2 27.900000 0 0\trobot status\t334.840327\t31.611878\t11.688100\t0.473510\t1.409771\t-43.611484\t0.243000\t0.103000\n\t\n15:27:21.7\tlog_raw\tgps_raw\t#DUALANTENNAHEADINGA,USB3,0,49.5,FINESTEERING,2107,282459.700,02000000,d426,15824;SOL_COMPUTED,L1_FLOAT,-1.000000000,51.464805603,-60.732208252,0.0,125.312278748,109.238609314,\"631T\",15,5,5,5,04,00,20,02*8c6ba398\n\tsystem status\tnormal 2 27.800000 0 0\trobot status\t334.932892\t31.501645\t11.690200\t0.530878\t1.273516\t-43.069908\t0.172000\t0.208000\n\t\n15:27:22.2\tlog_raw\tgps_raw\t\tsystem status\tnormal 2 27.800000 0 0\trobot status\t335.024250\t31.393243\t11.693300\t0.618880\t1.140669\t-42.504344\t0.315000\t0.003000\n\t\n15:27:22.7\tlog_raw\tgps_raw\t#DUALANTENNAHEADINGA,USB3,0,50.0,FINESTEERING,2107,282460.700,02000000,d426,15824;SOL_COMPUTED,L1_FLOAT,-1.000000000,54.102706909,-60.343048096,0.0,154.762100220,135.056198120,\"631T\",14,6,6,6,04,00,20,02*46d0133e\n\tsystem status\tnormal 2 27.800000 0 0\trobot status\t335.115501\t31.286887\t11.697300\t0.703371\t0.987593\t-41.900429\t0.340000\t-0.049000\n\t\n15:27:23.2\tlog_raw\tgps_raw\t#DUALANTENNAHEADINGA,USB3,0,51.0,FINESTEERING,2107,282461.200,02000000,d426,15824;SOL_COMPUTED,L1_FLOAT,-1.000000000,54.517234802,-56.248260498,0.0,106.436035156,86.120704651,\"631T\",12,6,6,6,04,00,20,02*7e772430\n\tsystem status\tnormal 2 27.900000 0 0\trobot status\t335.209302\t31.180862\t11.701100\t0.775091\t0.961138\t-41.275281\t0.272000\t0.073000\n\t\n15:27:23.7\tlog_raw\tgps_raw\t\tsystem status\tnormal 2 27.900000 0 0\trobot status\t335.303697\t31.077741\t11.705300\t0.704516\t0.992638\t-40.791290\t0.234000\t0.122000\n\t\n15:27:24.2\tlog_raw\tgps_raw\t#DUALANTENNAHEADINGA,USB3,0,53.0,FINESTEERING,2107,282462.200,02000000,d426,15824;SOL_COMPUTED,L1_FLOAT,-1.000000000,48.982975006,-50.048645020,0.0,87.434806824,84.797714233,\"631T\",12,6,6,6,04,00,20,02*0529a78d\n\tsystem status\tnormal 2 27.900000 0 0\trobot status\t335.397186\t30.975991\t11.708500\t0.778442\t1.152013\t-40.268913\t0.344000\t-0.033000\n\t\n15:27:24.7\tlog_raw\tgps_raw\t#DUALANTENNAHEADINGA,USB3,0,53.0,FINESTEERING,2107,282462.700,02000000,d426,15824;SOL_COMPUTED,L1_FLOAT,-1.000000000,49.117179871,-50.247711182,0.0,88.570533752,85.136001587,\"631T\",13,6,6,6,04,00,20,03*84c2d42f\n\tsystem status\tnormal 2 27.900000 0 0\trobot status\t335.492251\t30.875411\t11.709700\t0.846584\t1.253885\t-39.720481\t0.401000\t-0.126000\n\t\n15:27:25.2\tlog_raw\tgps_raw\t\tsystem status\tnormal 2 27.900000 0 0\trobot status\t335.589405\t30.773780\t11.711400\t0.996389\t1.221093\t-39.254231\t0.296000\t0.019000\n\t\n15:27:25.7\tlog_raw\tgps_raw\t#DUALANTENNAHEADINGA,USB3,0,54.0,FINESTEERING,2107,282463.700,02000000,d426,15824;SOL_COMPUTED,L1_FLOAT,-1.000000000,51.500408173,-54.802459717,0.0,108.538322449,83.711227417,\"631T\",15,6,6,6,04,00,20,02*3dcbf296\n\tsystem status\tnormal 2 27.900000 0 0\trobot status\t335.687735\t30.672815\t11.715500\t1.089393\t1.059128\t-38.904464\t0.378000\t-0.098000\n\t\n15:27:26.2\tlog_raw\tgps_raw\t\tsystem status\tnormal 2 27.900000 0 0\trobot status\t335.788200\t30.572927\t11.718900\t0.973821\t0.823982\t-38.619048\t0.229000\t0.112000\n\t\n15:27:26.7\tlog_raw\tgps_raw\t\tsystem status\tnormal 2 27.900000 0 0\trobot status\t335.889727\t30.473722\t11.722700\t0.783350\t0.748703\t-38.254622\t0.319000\t-0.023000\n\t\n15:27:27.2\tlog_raw\tgps_raw\t#DUALANTENNAHEADINGA,USB3,0,51.5,FINESTEERING,2107,282465.200,02000000,d426,15824;SOL_COMPUTED,NARROW_FLOAT,-1.000000000,56.702713013,-55.800750732,0.0,137.773193359,136.991073608,\"631T\",13,6,6,6,04,00,20,03*fede75fb\n\tsystem status\tnormal 2 27.900000 0 0\trobot status\t335.992554\t30.374065\t11.725200\t0.677806\t0.705023\t-37.867898\t0.253000\t0.069000\n\t\n15:27:27.7\tlog_raw\tgps_raw\t\tsystem status\tnormal 2 28.000000 0 0\trobot status\t336.093097\t30.275686\t11.727200\t0.721157\t0.813527\t-37.667177\t0.268000\t0.043000\n\t\n15:27:28.2\tlog_raw\tgps_raw\t#DUALANTENNAHEADINGA,USB3,0,49.5,FINESTEERING,2107,282466.200,02000000,d426,15824;SOL_COMPUTED,L1_FLOAT,-1.000000000,50.215934753,-52.944305420,0.0,107.166450500,95.447196960,\"631T\",15,6,6,6,04,00,20,02*0a3eeb82\n\tsystem status\tnormal 2 27.900000 0 0\trobot status\t336.195108\t30.177379\t11.729300\t0.657949\t0.838611\t-37.462360\t0.309000\t0.002000\n\t\n15:27:28.7\tlog_raw\tgps_raw\t\tsystem status\tnormal 2 27.900000 0 0\trobot status\t336.297254\t30.078353\t11.732100\t0.599757\t0.884777\t-37.192551\t0.282000\t0.047000\n\t\n15:27:29.2\tlog_raw\tgps_raw\t#INSPVAXA,USB3,0,49.5,FINESTEERING,2107,282467.250,02000000,471d,15824;INS_ALIGNMENT_COMPLETE,INS_RTKFIXED,37.37040027529,126.72463299399,11.7361,22.3000,-0.1940,0.1986,-0.0035,0.679971609,0.798971146,127.016292493,0.4355,0.2951,0.5412,0.1133,0.0928,0.0767,0.1368,0.1419,5.0947,0f000001,0*9f6381ee\n\tsystem status\tnormal 2 28.000000 0 0\trobot status\t336.410777\t29.967817\t11.736100\t0.679972\t0.798971\t-37.016292\t0.315000\t-0.029000\n\t\n15:27:29.7\tlog_raw\tgps_raw\t#DUALANTENNAHEADINGA,USB3,0,49.5,FINESTEERING,2107,282467.700,02000000,d426,15824;SOL_COMPUTED,L1_FLOAT,-1.000000000,52.617862701,-51.723999023,0.0,138.564620972,121.129493713,\"631T\",15,6,6,6,04,00,20,02*1b74d979\n\tsystem status\tnormal 2 27.900000 0 0\trobot status\t336.505364\t29.876903\t11.739100\t0.592253\t0.689267\t-36.832441\t0.416000\t-0.166000\n\t\n15:27:30.2\tlog_raw\tgps_raw\t#DUALANTENNAHEADINGA,USB3,0,52.5,FINESTEERING,2107,282468.200,02000000,d426,15824;SOL_COMPUTED,L1_FLOAT,-1.000000000,53.229724884,-52.106597900,0.0,138.289840698,109.253112793,\"631T\",16,6,6,6,04,00,20,02*279e2280\n\tsystem status\tnormal 2 27.900000 0 0\trobot status\t336.610566\t29.776814\t11.742100\t0.534085\t0.547387\t-36.490043\t0.204000\t0.150000\n\t\n15:27:30.7\tlog_raw\tgps_raw\t\tsystem status\tnormal 2 27.900000 0 0\trobot status\t336.715927\t29.678551\t11.745300\t0.369367\t0.545673\t-36.256468\t0.356000\t-0.063000\n\t\n15:27:31.2\tlog_raw\tgps_raw\t#DUALANTENNAHEADINGA,USB3,0,51.5,FINESTEERING,2107,282469.200,02000000,d426,15824;SOL_COMPUTED,L1_FLOAT,-1.000000000,53.708850861,-50.439453125,0.0,142.785049438,121.784484863,\"631T\",13,6,6,6,04,00,20,02*6a3bd9b0\n\tsystem status\tnormal 2 27.900000 0 0\trobot status\t336.820138\t29.579132\t11.748800\t0.383396\t0.624728\t-35.943977\t0.278000\t0.037000\n\t\n15:27:31.7\tlog_raw\tgps_raw\t\tsystem status\tnormal 2 27.900000 0 0\trobot status\t336.922467\t29.479680\t11.750900\t0.528246\t0.697261\t-35.518994\t0.289000\t0.036000\n\t\n15:27:32.2\tlog_raw\tgps_raw\t#DUALANTENNAHEADINGA,USB3,0,52.0,FINESTEERING,2107,282470.200,02000000,d426,15824;SOL_COMPUTED,L1_FLOAT,-1.000000000,64.190452576,-66.300750732,0.0,248.333297729,180.000000000,\"631T\",12,6,6,6,04,00,20,02*9fcca8a8\n\tsystem status\tnormal 2 27.900000 0 0\trobot status\t337.027393\t29.379378\t11.753100\t0.578367\t0.783667\t-35.037039\t0.252000\t0.109000\n\t\n15:27:32.7\tlog_raw\tgps_raw\t#INSPVAXA,USB3,0,52.0,FINESTEERING,2107,282470.750,02000000,471d,15824;INS_ALIGNMENT_COMPLETE,INS_RTKFIXED,37.37039399952,126.72464125042,11.7560,22.3000,-0.1944,0.2055,0.0095,0.556382070,0.833580794,124.571491117,0.4368,0.2954,0.5421,0.1138,0.0931,0.0768,0.1367,0.1417,5.0972,0f000001,0*6c9732d6\n\tsystem status\tnormal 2 27.900000 0 0\trobot status\t337.142118\t29.271273\t11.756000\t0.556382\t0.833581\t-34.571491\t0.225000\t0.137000\n\t\n15:27:33.2\tlog_raw\tgps_raw\t#DUALANTENNAHEADINGA,USB3,0,53.0,FINESTEERING,2107,282471.200,02000000,d426,15824;SOL_COMPUTED,NARROW_FLOAT,-1.000000000,77.375328064,-72.297668457,0.0,360.000000000,180.000000000,\"631T\",16,6,6,6,04,00,20,03*599578cb\n\tsystem status\tnormal 2 27.900000 0 0\trobot status\t337.237728\t29.185606\t11.760300\t0.323421\t0.925846\t-34.068444\t0.315000\t0.005000\n\t\n15:27:33.7\tlog_raw\tgps_raw\t\tsystem status\tnormal 2 27.800000 0 0\trobot status\t337.346243\t29.091340\t11.764900\t0.186325\t0.920086\t-33.487522\t0.249000\t0.097000\n\t\n15:27:34.2\tlog_raw\tgps_raw\t
